vi "SensorIntensidad_Final_Temp.vi"() -> ()   [LabVIEW 2024]
uses:
  <vilib>/userDefined/High Color/IMAQdx.ctl
  <vilib>/vision/driver/IMAQdx.llb/IMAQdx Buffer Number Mode.ctl
  <vilib>/vision/driver/IMAQdx.llb/IMAQdx Acquisition Mode.ctl
  <vilib>/express/express shared/transition.llb/Dynamic To Waveform Array.vi
  <vilib>/express/express signal manip/GetorSetDDTAttributes/Set DDT Attributes/SetT0.vi
  <vilib>/express/express shared/transition.llb/Waveform Array To Dynamic.vi
  <vilib>/express/express signal manip/GetorSetDDTAttributes/Set DDT Attributes/Set DDT Properties.xnode
  <vilib>/vision/driver/NI_Vision_Acquisition_Software.lvlib
  <vilib>/vision/NI_Vision_Development_Module.lvlib
  <instrlib>/Arduino UNO/Arduino UNO.lvlib
panel:
  out "Temperature Heater":dbl
  out "Temperature 2":string
  out "Temperature Ambient":dbl
  out "Temperature":string
  in  "VISA Arduino":refnum<visa-resource-name>
  out "XY Graph":cluster{"Run Time (ms)":u32, "IM":sgl}[](graph)
  out "IM":sgl
  out "Rec":T1 {"Rotation" format="%.2f"; "Left" scale=0.0..1024.0; "Right" scale=0.0..1024.0}
  in  "Buffer Mode":T2
  in  "Cancel Button":bool
  out "frame rate (fps)":u32
  out "Run Time (ms)":u32
  out "ms timer":u32
  in  "Session In":T3
  out "Image":T4(plugin-control)
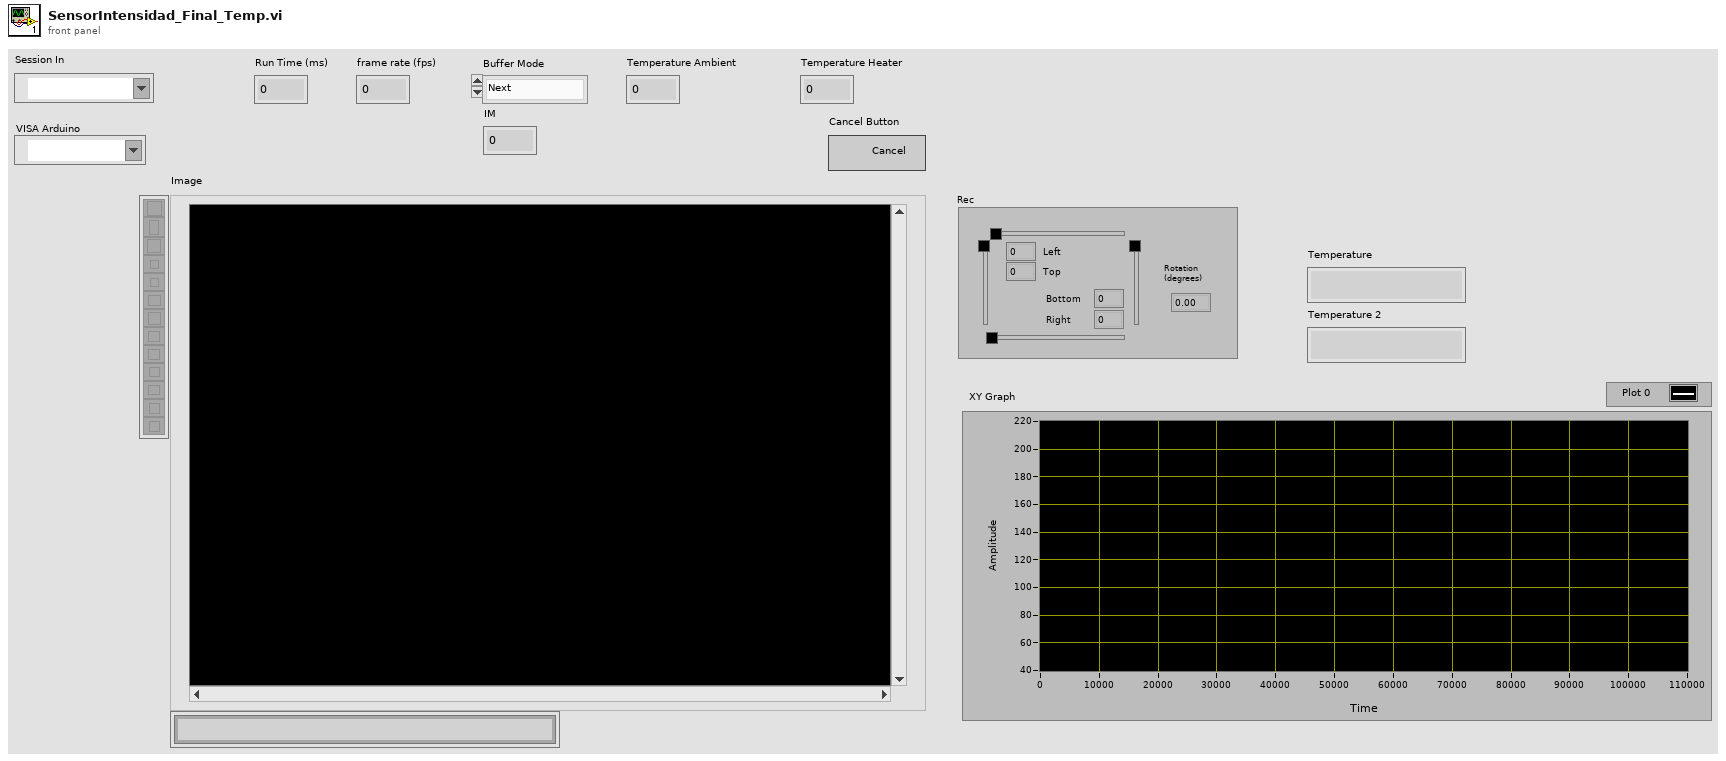
[diagram p1: front panel]
types:
  T1 = typedef "IMAQ Rectangle" = cluster{"Left":i32, "Top":i32, "Right":i32, "Bottom":i32, "Rotation":dbl}
  T2 = typedef "NI_Vision_Acquisition_Software.lvlib/IMAQdx Buffer Number Mode.ctl" = enum32{"Next", "Last", "Buffer Number", "Every", "Last New"}
  T3 = typedef "IMAQdx.ctl" = refnum<k21>
  T4 = typedef "IMAQ Image.ctl" = refnum<image>
  T5 = typedef "Image Type" = u32
  T6 = typedef "NI_Vision_Acquisition_Software.lvlib/IMAQdx Acquisition Mode.ctl" = enum32{"One Shot", "Continuous"}
  T7 = cluster{"Global Rectangle":i32[], "Contours":cluster{"Contour Type":u32, "ROI Type":u32, "Points":i32[]}[]}
  T8 = cluster{"Mean Intensity":sgl, "Standard  Deviation":sgl, "Minimum Intensity":sgl, "Maximum Intensity":sgl}
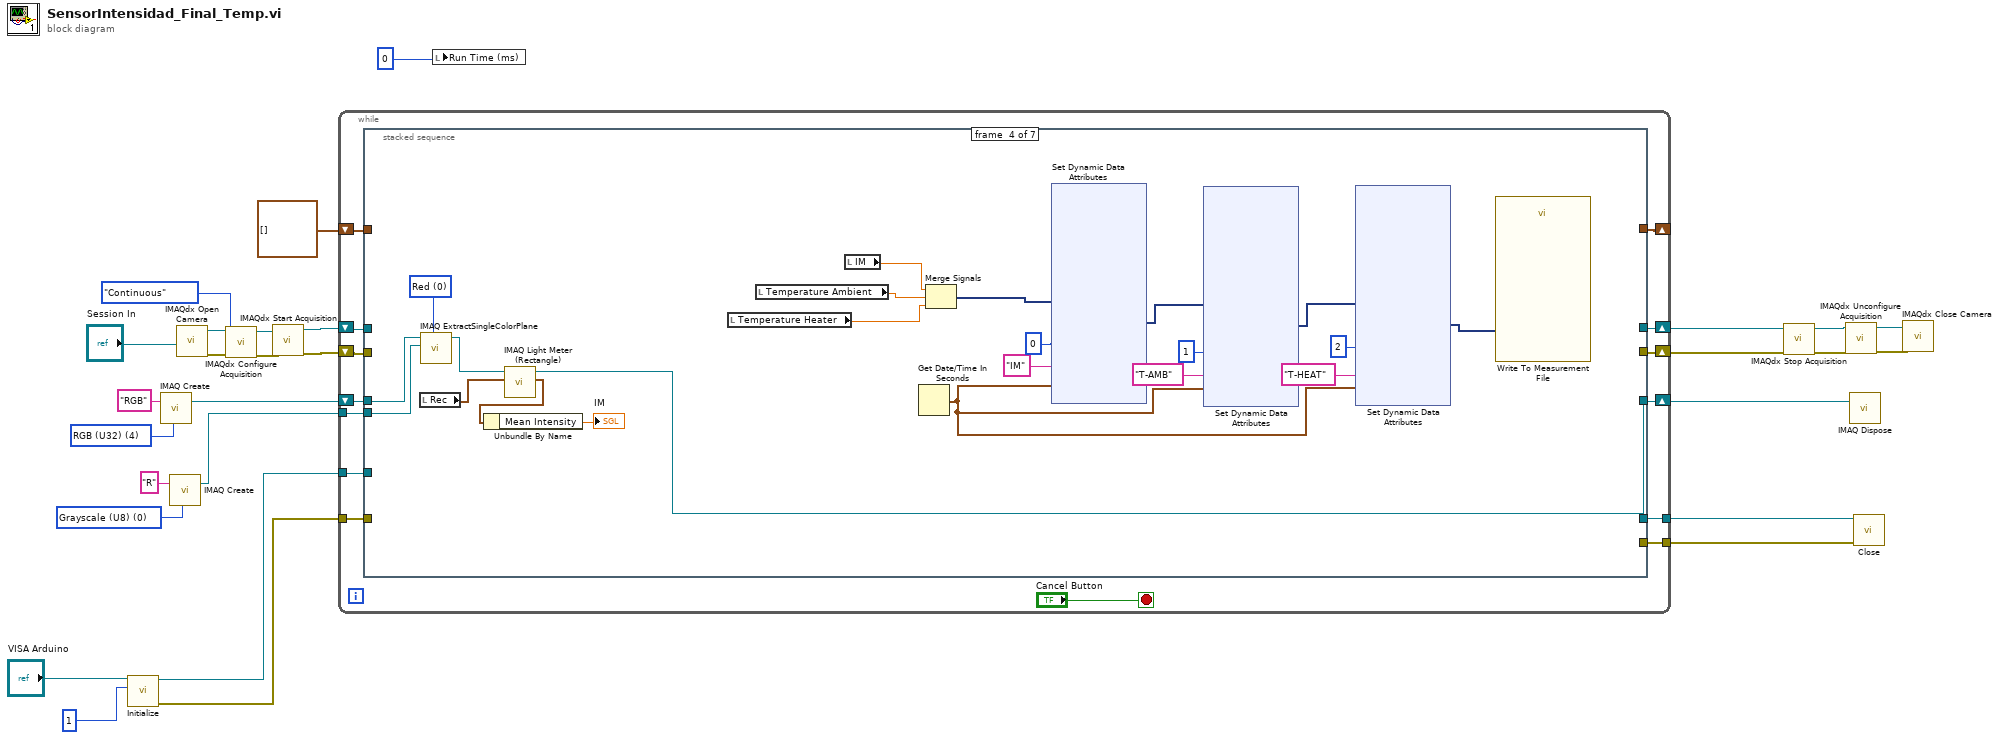
[diagram p0: block diagram]
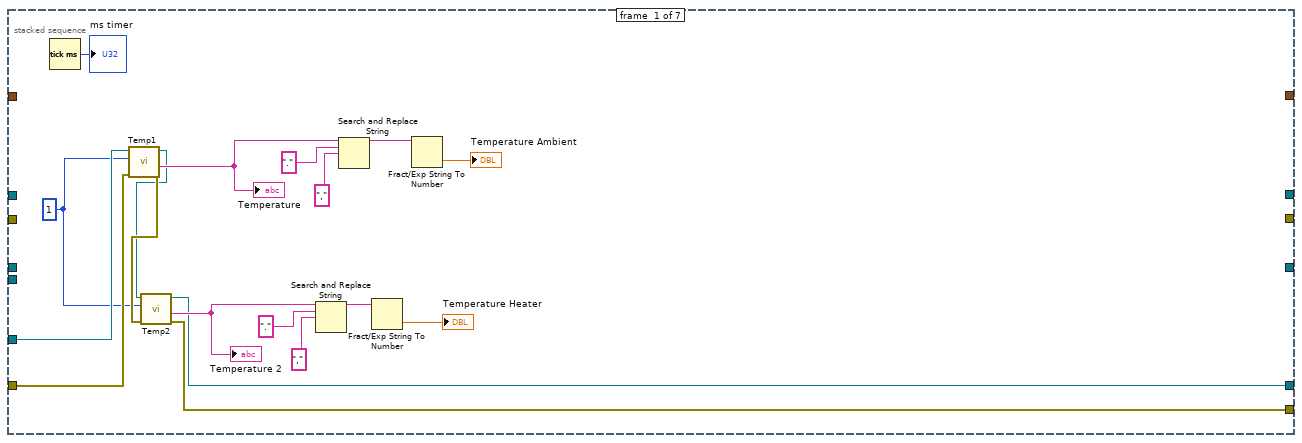
[diagram p2: hidden frame]
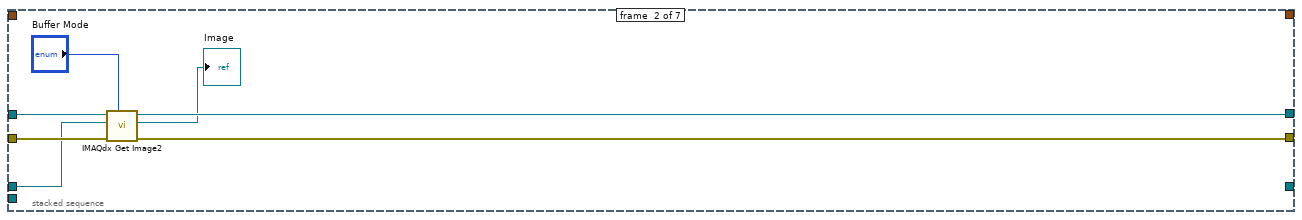
[diagram p3: hidden frame]
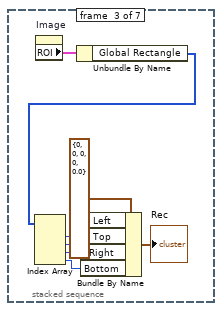
[diagram p4: hidden frame]
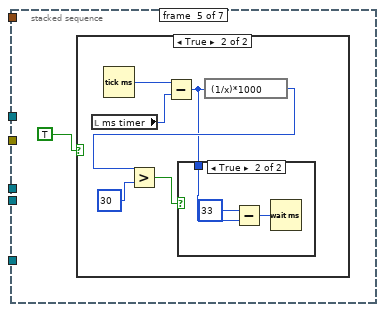
[diagram p5: hidden frame]
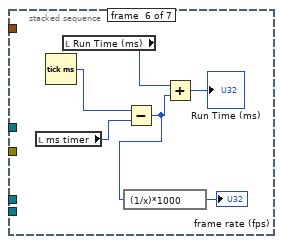
[diagram p8: hidden frame]
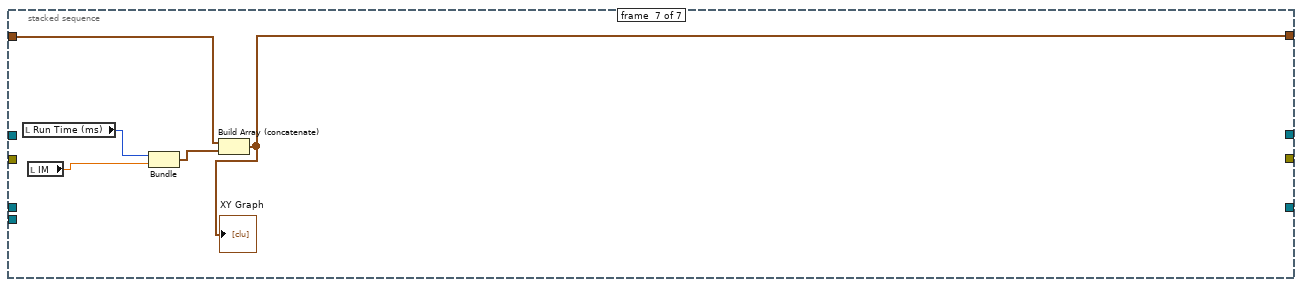
[diagram p9: hidden frame]
diagram:
  w8 = T5 0 items=["Grayscale (U8)", "Grayscale (I16)", "Grayscale (SGL)", "Complex (CSG)", "RGB (U32)", "HSL (U32)", "RGB (U64)", "Grayscale (U16)"] ("Image Type")
  w18 = T5 4 items=["Grayscale (U8)", "Grayscale (I16)", "Grayscale (SGL)", "Complex (CSG)", "RGB (U32)", "HSL (U32)", "RGB (U64)", "Grayscale (U16)"] ("Image Type")
  n1 = call <instrlib>:"Initialize.vi"("Address"=1, "VISA resource name"="VISA Arduino") -> ("error IO"=w4:errorcluster, "VISA resource name out"=w3:refnum<visa-resource-name>)  [unwired: 7 in, 1 out]
  n2 = call "IMAQ Create"("Image Name"="RGB", "Image Type"=w18) -> ("New Image"=w17:T4)  [unwired: 3 in, 1 out]
  n3 = call "IMAQ Create"("Image Name"="R", "Image Type"=w8) -> ("New Image"=w7:T4)  [unwired: 3 in, 1 out]
  n4 = call <vilib>:"IMAQdx Open Camera.vi"("Session In"="Session In") -> ("error out"=w28:errorcluster, "Session Out"=w29:T3)  [unwired: 9 in]
  n5 = call <vilib>:"IMAQdx Configure Acquisition.vi"("error in"=w28, "Continuous?"=IMAQdx_Acquisition_Mode."Continuous", "Session In"=w29) -> ("error out"=w26:errorcluster, "Session Out"=w27:T3)  [unwired: 7 in]
  n6 = call <vilib>:"IMAQdx Start Acquisition.vi"("error in"=w26, "Session In"=w27) -> ("error out"=w24:errorcluster, "Session Out"=w25:T3)  [unwired: 8 in]
  n7 = while {
    shift-right: [w40] -> w16
    shift-left: w25 -> [w43]
    shift-right: [w39] -> w15
    shift-left: w24 -> [w42]
    shift-right: [w37] -> _
    shift-left: cluster{"Run Time (ms)":u32, "IM":sgl}[] [] -> [w36]
    shift-right: [w35] -> w10
    shift-left: w17 -> [w41]
    tunnel: w7 -> [w34]
    tunnel: w4 -> [w33]
    tunnel: w3 -> [w32]
    tunnel: [w31] -> w2
    tunnel: [w30] -> w1
    stop <- "Cancel Button" stop-if-true
    n8 = stacked-sequence {
      tunnel: w43 -> [_ w68 _ _ _ _ _]
      tunnel: w42 -> [_ w67 _ _ _ _ _]
      tunnel: w41 -> [_ w66 _ w95 _ _ _]
      tunnel: [_ w65 _ _ _ _ _] -> w40
      tunnel: [_ w64 _ _ _ _ _] -> w39
      tunnel: [_ _ _ _ _ _ w168] -> w37
      tunnel: w36 -> [_ _ _ _ _ _ w167]
      tunnel: [_ _ _ w94 _ _ _] -> w35
      tunnel: w34 -> [_ _ _ w92 _ _ _]
      tunnel: w33 -> [w48 _ _ _ _ _ _]
      tunnel: w32 -> [w47 _ _ _ _ _ _]
      tunnel: [w46 _ _ _ _ _ _] -> w31
      tunnel: [w45 _ _ _ _ _ _] -> w30
      frame #0 {
        w44 = 1
        n9 = Tick Count (ms)() -> (millisecond timer value=→"ms timer":u32)
        n10 = call <instrlib>:"Temp1.vi"("error in (no error)"=w48, "Address"=w44, "VISA resource name"=w47) -> ("error IO"=w55:errorcluster, "Pressure"=w56:string, "VISA resource name out"=w54:refnum<visa-resource-name>)  [unwired: 6 in]
        "Temperature" <- w56
        n11 = call <instrlib>:"Temp2.vi"("error in (no error)"=w55, "Address"=w44, "VISA resource name"=w54) -> ("error IO"=w46:errorcluster, "Pressure"=w50:string, "VISA resource name out"=w45:refnum<visa-resource-name>)  [unwired: 6 in]
        "Temperature 2" <- w50
        n12 = Search and Replace String(input string=w50, search string=".", replace string=",") -> (result string=w51:string)  [unwired: 5 in, 3 out]
        n13 = Search and Replace String(input string=w56, search string=".", replace string=",") -> (result string=w58:string)  [unwired: 5 in, 3 out]
        n14 = Fract/Exp String To Number(string=w51) -> (number=→"Temperature Heater":dbl)  [unwired: 3 in, 1 out]
        n15 = Fract/Exp String To Number(string=w58) -> (number=→"Temperature Ambient":dbl)  [unwired: 3 in, 1 out]
      }
      frame #1 {
        n16 = call <vilib>:"IMAQdx Get Image2.vi"("Buffer Number Mode (Next)"="Buffer Mode", "error in"=w67, "Image In"=w66, "Session In"=w68) -> ("error out"=w64:errorcluster, "Image Out"=→"Image":T4, "Session Out"=w65:T3)  [unwired: 4 in, 1 out]
      }
      frame #2 {
        n17 = property on="Image" class="ImageControl"() -> ("ROI"=w76:T7)  [unwired: 2 in, 2 out]
        n18 = Unbundle By Name(w76) -> ("Global Rectangle"=w69:i32[])
        n19 = Index Array(array=w69) -> (element #1=w74:i32, element #2=w73:i32, element #3=w72:i32, element #4=w71:i32)  [unwired: 4 in]
        n20 = Bundle By Name(cluster=T1 {"Left"=0, "Top"=0, "Right"=0, "Bottom"=0, "Rotation"=0.0} ("Rectangle"), "Left"=w74, "Top"=w73, "Right"=w72, "Bottom"=w71) -> (→"Rec":T1)
      }
      frame #3 {
        w93 = 0 items=["Red", "Green", "Blue", "Hue", "Saturation", "Luminance", "Value", "Intensity"] ("Color Plane")
        n21 = local read "Rec"() -> (w98:T1)
        n22 = call "IMAQ ExtractSingleColorPlane"("Color Plane"=w93, "Image Dst"=w92, "Image Src"=w95) -> ("Image Dst Out"=w87:T4)  [unwired: 7 in, 1 out]
        n23 = call "IMAQ Light Meter (Rectangle)"("Rectangle"=w98, "Image"=w87) -> ("Gray Level Intensities"=w97:T8, "Image Out"=w94:T4)  [unwired: 5 in, 3 out]
        n24 = Unbundle By Name(w97) -> ("Mean Intensity"=→"IM":sgl)
        n25 = local read "Temperature Heater"() -> (w77:dbl)
        n26 = local read "Temperature Ambient"() -> (w78:dbl)
        n27 = local read "IM"() -> (w88:sgl)
        n28 = Get Date/Time In Seconds() -> (seconds since 1Jan1904=w84:timestamp)
        n29 = Merge Signals(w88, w78, w77) -> (w91:dynamicdata)
        n30 = xnode "Set Dynamic Data Attributes"("Signals In"=w91, "Signal Index"=0, "Signal Name"="IM", "Timestamp"=w84) -> ("Signals Out"=w81:dynamicdata)  [unwired: 1 in, 1 out]
        n31 = xnode "Set Dynamic Data Attributes"("Signals In"=w81, "Signal Index"=1, "Signal Name"="T-AMB", "Timestamp"=w84) -> ("Signals Out"=w80:dynamicdata)  [unwired: 1 in, 1 out]
        n32 = xnode "Set Dynamic Data Attributes"("Signals In"=w80, "Signal Index"=2, "Signal Name"="T-HEAT", "Timestamp"=w84) -> ("Signals Out"=w79:dynamicdata)  [unwired: 1 in, 1 out]
        n33 = call "Write To Measurement File"("Signals"=w79) -> ()  [unwired: 16 in, 3 out]
      }
      frame #4 {
        n34 = case shown="True" TRUE {
          frame False {
          }
          frame True {
            n35 = local read "ms timer"() -> (w155:u32)
            n36 = Tick Count (ms)() -> (millisecond timer value=w156:u32)
            n37 = Subtract(x=w156, y=w155) -> (x-y=w152:u32)
            n38 = expression code="(1/x)*1000"(w152) -> (w154:u32)
            n39 = Greater?(x=w154, y=u32 30) -> (0:w151:bool)
            n40 = case shown="True" w151 {
              tunnel: w152 -> [_ w159]
              frame False {
              }
              frame True {
                n41 = Subtract(x=u32 33, y=w159) -> (x-y=w157:u32)
                n42 = Wait (ms)(milliseconds to wait=w157) -> ()  [unwired: 1 out]
              }
            }
          }
        }
      }
      frame #5 {
        n43 = local read "ms timer"() -> (w165:u32)
        n44 = Tick Count (ms)() -> (millisecond timer value=w164:u32)
        n45 = local read "Run Time (ms)"() -> (w162:u32)
        n46 = Subtract(x=w164, y=w165) -> (x-y=w161:u32)
        n47 = expression code="(1/x)*1000"(w161) -> (→"frame rate (fps)":u32)
        n48 = Add(x=w162, y=w161) -> (x+y=→"Run Time (ms)":u32)
      }
      frame #6 {
        n49 = local read "Run Time (ms)"() -> (w170:u32)
        n50 = local read "IM"() -> (w166:sgl)
        n51 = Bundle("Run Time (ms)"=w170, "IM"=w166) -> (w169:cluster{"Run Time (ms)":u32, "IM":sgl})  [unwired: 1 in]
        n52 = Build Array (concatenate)(w167, w169) -> (w168:cluster{"Run Time (ms)":u32, "IM":sgl}[])
        "XY Graph" <- w168
      }
    }
  }
  n53 = local write "Run Time (ms)"(u32 0 ("Run Time")) -> ()
  n54 = call <vilib>:"IMAQdx Stop Acquisition.vi"("error in"=w15, "Session In"=w16) -> ("error out"=w22:errorcluster, "Session Out"=w23:T3)  [unwired: 8 in]
  n55 = call <vilib>:"IMAQdx Unconfigure Acquisition.vi"("error in"=w22, "Session In"=w23) -> ("error out"=w21:errorcluster, "Session Out"=w20:T3)  [unwired: 8 in]
  n56 = call "IMAQ Dispose"("Image"=w10) -> ()  [unwired: 5 in, 1 out]
  n57 = call <instrlib>:"Close.vi"("error in (no error)"=w2, "VISA resource name"=w1) -> ()  [unwired: 9 in, 1 out]
  n58 = call <vilib>:"IMAQdx Close Camera.vi"("error in"=w21, "Session In"=w20) -> ()  [unwired: 9 in, 1 out]
